vi "Cal RowNum(SubVI).vi"(5 "Width":i16, 7 "curCol":i16, 8 "Ready For Input":bool, 9 "EndOfImage":bool, 10 "curRow":i16, 11 "EOL":bool) -> (3 "nextRow":i16)   [LabVIEW 2016]
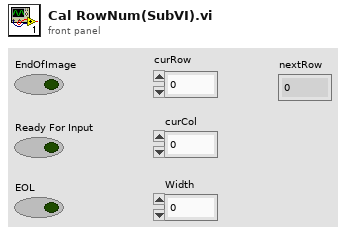
[diagram p1: front panel]
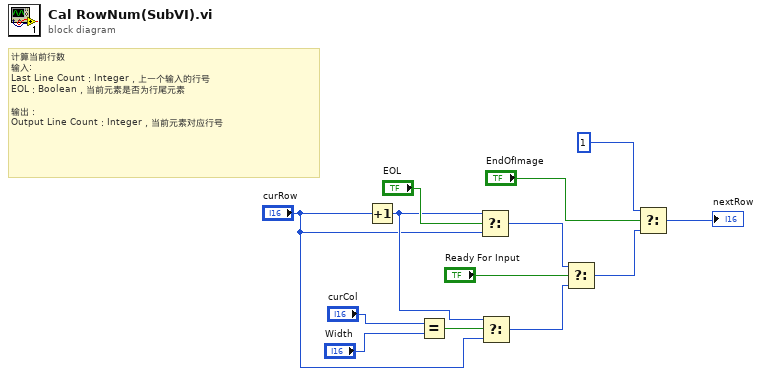
[diagram p0: block diagram]
diagram:
  # "计算当前行数\n输入:\nLast Line Count：Integer，上一个输入的行号\nEOL：Boolean，当前元素是否为行尾元素\n\n输出：\nOutput Line Count：Integer，当前元素对应行号"
  n1 = Increment(x="curRow") -> (x+1=w7:i16)
  n2 = Equal?(x="curCol", y="Width") -> (x = y?=w8:bool)
  n3 = Select(t=w7, s="EOL", f="curRow") -> (s? t:f=w5:i16)
  n4 = Select(t=w7, s=w8, f="curRow") -> (s? t:f=w9:i16)
  n5 = Select(t=w5, s="Ready For Input", f=w9) -> (s? t:f=w4:i16)
  n6 = Select(t=i16 1, s="EndOfImage", f=w4) -> (s? t:f=→"nextRow":i16)
